vi "PFI-28000-Chan-Bridge_Set Bypass.vi"(8 "error in (no error)":errorcluster, 10 "Bypass":bool, 11 "PFI-28000-Chan-Bridge in":refnum<class "PFI-28000-Chan-Bridge.lvclass">) -> (0 "error out":errorcluster, 3 "PFI-28000-Chan-Bridge out":refnum<class "PFI-28000-Chan-Bridge.lvclass">)   [LabVIEW 2017, in "PFI-28000-Chan-Bridge.lvclass"]
uses:
  PFI-28000-Chan-Bridge.lvclass
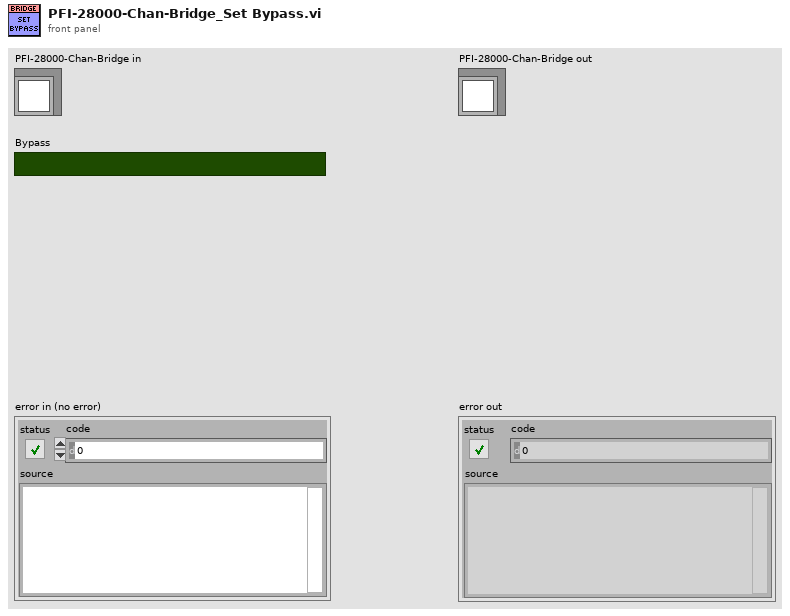
[diagram p1: front panel]
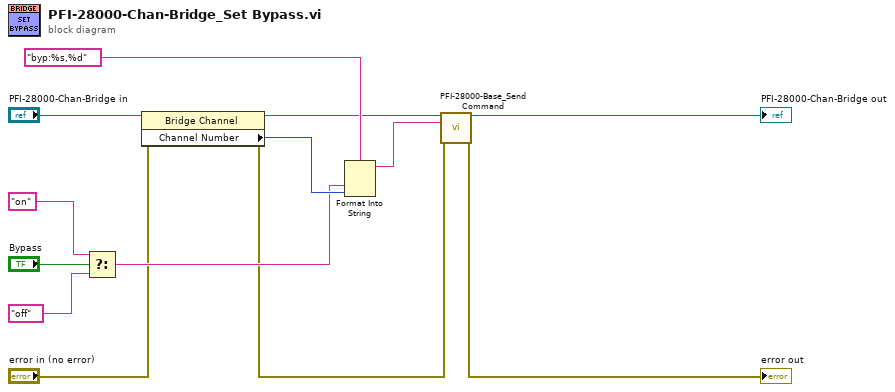
[diagram p0: block diagram]
diagram:
  n1 = Select(t="on" ("empty string"), s="Bypass", f="off" ("empty string")) -> (s? t:f=w7:string)
  n2 = property class="Bridge Channel"(reference="PFI-28000-Chan-Bridge in", error in="error in (no error)") -> (reference out=w5:refnum<class "PFI-28000-Chan-Bridge.lvclass">, error out=w2:errorcluster, "Channel Number"=w8:i32)
  n3 = Format Into String(format string="byp:%s,%d" ("empty string"), w7, w8) -> (resulting string=w3:string)  [unwired: 2 in, 1 out]
  n4 = call-dynamic "PFI-28000-Base_Send Command.vi"("PFI-28000-Base in"=w5, "Command"=w3, "error in (no error)"=w2) -> ("PFI-28000-Base out"=→"PFI-28000-Chan-Bridge out":refnum<class "PFI-28000-Chan-Bridge.lvclass">, "error out"=→"error out":errorcluster)  [unwired: 11 in]
